vi "Export Plot.vi"(8 "Path 2":path, 9 "String":string="FFT_%m.%d.%Y_%H.%M", 10 "Array":string[](array[string]), 11 "File Format":enum32{"BMP", "EPS", "EMF", "PICT"}(ring)) -> (0 "Canceled?":bool, 3 "Path":path)   [LabVIEW 2018]
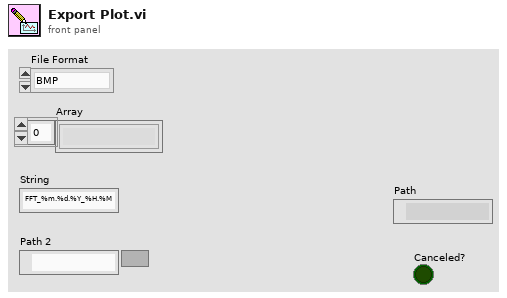
[diagram p1: front panel]
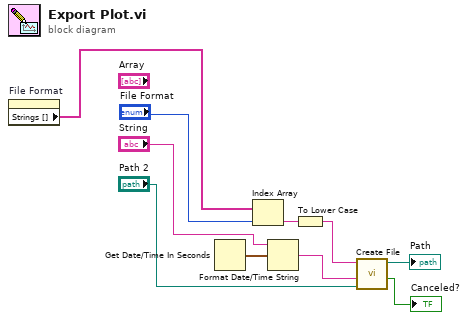
[diagram p0: block diagram]
diagram:
  n1 = property on="File Format" class="Enum (strict)"() -> ("Strings []"=w2:string[])  [unwired: 2 in, 2 out]
  n2 = Get Date/Time In Seconds() -> (seconds since 1Jan1904=w9:timestamp)
  n3 = Index Array(array=w2, index="File Format") -> (element=w8:string)
  n4 = Format Date/Time String(time format string (%c)="String", seconds (now)=w9) -> (date/time string=w4:string)  [unwired: 1 in]
  n5 = To Lower Case(string=w8) -> (all lower case string=w7:string)
  n6 = call "Create File.vi"("Start Path"="Path 2", "Default File Name"=w4, "File Extension"=w7) -> ("canceled?"=→"Canceled?":bool, "File Path"=→"Path":path)  [unwired: 7 in]
